vi "curves_statistics.vi"(11 "T1_curves":T1(array[cluster])) -> (0 "stdev_curve":cluster{"dark_time_us":dbl[], "PL_signal":dbl[]}, 1 "stdev":dbl[](array[numeric]), 2 "mean_curve":cluster{"dark_time_us":dbl[], "PL_signal":dbl[]}, 3 "mean":dbl[](array[numeric]), 4 "mean_stdev":dbl format="%0.2f")   [LabVIEW 2014]
uses:
  <vilib>/Analysis/NI_AALBase.lvlib
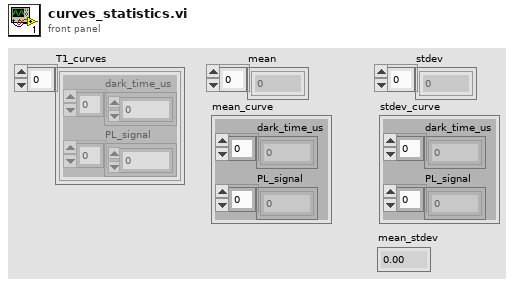
[diagram p1: front panel]
types:
  T1 = cluster{"dark_time_us":dbl[], "PL_signal":dbl[]}[]
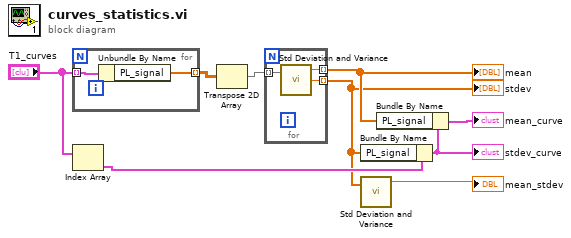
[diagram p0: block diagram]
diagram:
  n1 = for {
    tunnel: "T1_curves" -> [w10] mode=indexing
    tunnel: [w11] -> w8 mode=indexing
    n2 = Unbundle By Name(w10) -> ("PL_signal"=w11:dbl[])
  }
  n3 = Index Array(array="T1_curves") -> (element=w5:cluster{"dark_time_us":dbl[], "PL_signal":dbl[]})  [unwired: 1 in]
  n4 = Transpose 2D Array(2D array=w8) -> (transposed array=w9:dbl[][])
  n5 = for {
    tunnel: w9 -> [w14] mode=indexing
    tunnel: [w13] -> w7 mode=indexing
    tunnel: [w12] -> w2 mode=indexing
    n6 = call <vilib>:"Std Deviation and Variance.vi"("X"=w14) -> ("mean"=w13:dbl, "standard deviation"=w12:dbl)  [unwired: 1 in, 1 out]
  }
  "mean" <- w7
  "stdev" <- w2
  n7 = Bundle By Name(cluster=w5, "PL_signal"=w2) -> (w4:cluster{"dark_time_us":dbl[], "PL_signal":dbl[]})
  "stdev_curve" <- w4
  n8 = call <vilib>:"Std Deviation and Variance.vi"("X"=w2) -> ("mean"=→"mean_stdev":dbl)  [unwired: 1 in, 2 out]
  n9 = Bundle By Name(cluster=w4, "PL_signal"=w7) -> (→"mean_curve":cluster{"dark_time_us":dbl[], "PL_signal":dbl[]})
